vi "Climber_Hardware_Loop.vi"   [LabVIEW 2020]
uses:
  <vilib>/Rock Robotics/WPI/ThirdParty/Phoenix-LabVIEW/Motor Controller/Controls/CTRE_Phoenix_MotorControl_ControlMode.ctl
  Climber_Hardware_Globals.vi
  Globals/Climber_Globals.vi
  <vilib>/Rock Robotics/WPI/Solenoid/WPI_SolenoidSetEnum.vi
types:
  T1 = typedef "WPI_MotorControlDeviceRef.ctl" = cluster{"DeviceStatus":errorcluster, "Type":T2, "PWM":cluster{"PWM Channel":T3, "DeadBand":T4}, "CAN":cluster{"Device Number":u8, "SetOutput VI Ref":variant, "GetOutput VI Ref":variant, "Enable VI Ref":variant, "Disable VI Ref":variant, "Data":variant}, "Invert":bool, "DIO PWM":cluster{"PWM \"Enable\" Channel":T3, "DIOChannel":T5, "PWM Rate":dbl}}
  T2 = typedef "WPI_MotorControlType.ctl" = enum16{"PWM", "CAN", "DIO PWM"}
  T3 = typedef "FPGA_DIOPWMChannel.ctl" = enum8{"PWM 0", "PWM 1", "PWM 2", "PWM 3", "PWM 4", "PWM 5", "PWM 6", "PWM 7", "PWM 8", "PWM 9", "PWM MXP 0", "PWM MXP 1", "PWM MXP 2", "PWM MXP 3", "PWM MXP 4", "PWM MXP 5", "PWM MXP 6", "PWM MXP 7", "PWM MXP 8", "PWM MXP 9", "Invalid"}
  T4 = typedef "WPI_PWMDeadband.ctl" = cluster{"Name":string, "maxPositivePwm":i32, "minPositivePwm":i32, "centerPwm":i32, "maxNegativePwm":i32, "minNegativePwm":i32, "angularRange":u16}
  T5 = typedef "FPGA_DIOChannel.ctl" = enum8{"DIO 0", "DIO 1", "DIO 2", "DIO 3", "DIO 4", "DIO 5", "DIO 6", "DIO 7", "DIO 8", "DIO 9", "DIO MXP 0", "DIO MXP 1", "DIO MXP 2", "DIO MXP 3", "DIO MXP 4", "DIO MXP 5", "DIO MXP 6", "DIO MXP 7", "DIO MXP 8", "DIO MXP 9", "DIO MXP 10", "DIO MXP 11", "DIO MXP 12", "DIO MXP 13", "DIO MXP 14", "DIO MXP 15", "SPI Port CS1", "SPI Port CS2", "SPI Port CS3", "SPI Port MISO", "SPI Port MOSI", "Invalid"}
  T6 = typedef "WPI_SolenoidDevRef.ctl" = cluster{"DevStatus":errorcluster, "Pneumatics Control Module":u8, "Forward Solenoid Channel":T7, "Reverse Solenoid Channel":T7}
  T7 = typedef "WPI_SolenoidChannel.ctl" = enum8{"Solenoid 0", "Solenoid 1", "Solenoid 2", "Solenoid 3", "Solenoid 4", "Solenoid 5", "Solenoid 6", "Solenoid 7", "Solenoid 8", "Solenoid 9", "Solenoid 10", "Solenoid 11", "Solenoid 12", "Solenoid 13", "Solenoid 14", "Solenoid 15", "Invalid"}
  T8 = typedef "CTRE_Phoenix_MotorControl_ControlMode.ctl" = u16
  T9 = typedef "WPI_SolenoidValue.ctl" = enum16{"No_Change", "Off", "On", "Forward", "Reverse"}
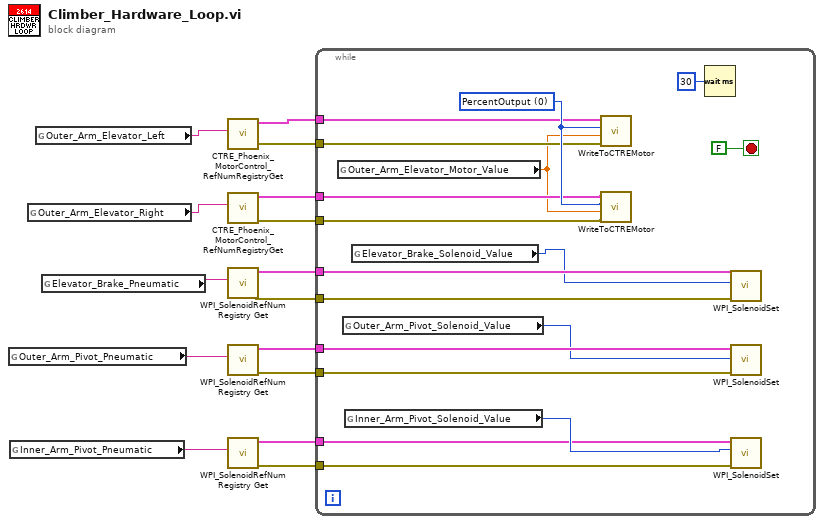
[diagram p0: block diagram]
diagram:
  n1 = global read "Climber_Hardware_Globals.vi" "Outer_Arm_Pivot_Pneumatic"() -> (w4:string)
  n2 = global read "Climber_Hardware_Globals.vi" "Inner_Arm_Pivot_Pneumatic"() -> (w3:string)
  n3 = global read "Climber_Hardware_Globals.vi" "Outer_Arm_Elevator_Right"() -> (w8:string)
  n4 = global read "Climber_Hardware_Globals.vi" "Outer_Arm_Elevator_Left"() -> (w7:string)
  n5 = global read "Climber_Hardware_Globals.vi" "Elevator_Brake_Pneumatic"() -> (w9:string)
  n6 = call <vilib>:"CTRE_Phoenix_MotorControl_RefNumRegistryGet.vi"("refnum name"=w7) -> ("error out"=w13:errorcluster, "PhoenixMotorControlDevRef"=w12:T1)  [unwired: 9 in]
  n7 = call <vilib>:"CTRE_Phoenix_MotorControl_RefNumRegistryGet.vi"("refnum name"=w8) -> ("error out"=w15:errorcluster, "PhoenixMotorControlDevRef"=w14:T1)  [unwired: 9 in]
  n8 = call <vilib>:"WPI_SolenoidRefNum Registry Get.vi"("refnum name"=w9) -> ("error out"=w11:errorcluster, "SolenoidDevRef"=w10:T6)  [unwired: 9 in]
  n9 = call <vilib>:"WPI_SolenoidRefNum Registry Get.vi"("refnum name"=w4) -> ("error out"=w5:errorcluster, "SolenoidDevRef"=w6:T6)  [unwired: 9 in]
  n10 = call <vilib>:"WPI_SolenoidRefNum Registry Get.vi"("refnum name"=w3) -> ("error out"=w2:errorcluster, "SolenoidDevRef"=w1:T6)  [unwired: 9 in]
  n11 = while {
    tunnel: w10 -> [w30]
    tunnel: w11 -> [w29]
    tunnel: w12 -> [w25]
    tunnel: w13 -> [w24]
    tunnel: w14 -> [w23]
    tunnel: w15 -> [w21]
    tunnel: w6 -> [w28]
    tunnel: w5 -> [w27]
    tunnel: w1 -> [w16]
    tunnel: w2 -> [w17]
    stop <- FALSE stop-if-true
    w26 = T8 0 items=["PercentOutput"=0, "Position"=1, "Velocity"=2, "Current"=3, "Follower"=5, "MotionProfile"=6, "MotionMagic"=7, "MotionProfileArc"=10, "Disabled"=15] ("Control Mode")
    n12 = global read "Climber_Globals.vi" "Outer_Arm_Elevator_Motor_Value"() -> (w22:dbl)
    n13 = global read "Climber_Globals.vi" "Outer_Arm_Pivot_Solenoid_Value"() -> (w19:T9)
    n14 = global read "Climber_Globals.vi" "Inner_Arm_Pivot_Solenoid_Value"() -> (w18:T9)
    n15 = global read "Climber_Globals.vi" "Elevator_Brake_Solenoid_Value"() -> (w20:T9)
    n16 = call "WriteToCTREMotor.vi"("error in (no error)"=w24, "Motor_Value"=w22, "Control Mode"=w26, "PhoenixMotorControlDevRef"=w25) -> ()  [unwired: 8 in]
    n17 = call "WriteToCTREMotor.vi"("error in (no error)"=w21, "Motor_Value"=w22, "Control Mode"=w26, "PhoenixMotorControlDevRef"=w23) -> ()  [unwired: 8 in]
    n18 = Wait (ms)(milliseconds to wait=u32 30) -> ()  [unwired: 1 out]
    n19 = call-poly <vilib>:"WPI_SolenoidSet.vi"("error in (no error)"=w29, "Value"=w20, "SolenoidDevRef"=w30) -> ()  [unwired: 7 in, 2 out]
    n20 = call-poly <vilib>:"WPI_SolenoidSet.vi"("error in (no error)"=w27, "Value"=w19, "SolenoidDevRef"=w28) -> ()  [unwired: 7 in, 2 out]
    n21 = call-poly <vilib>:"WPI_SolenoidSet.vi"("error in (no error)"=w17, "Value"=w18, "SolenoidDevRef"=w16) -> ()  [unwired: 7 in, 2 out]
  }
